vi "Multiply Quaternion by Quaternion.vi"(1 "y":T1, 2 "quaternion":T1) -> (0 "product":T1)   [LabVIEW 2017, in "NI_Kinematics.lvlib"]
doc: "Returns the <B>product</B> of two quaternions or a quaternion and a scalar number. Wire data to the <B>y</B> input to determine the polymorphic instance to use or manually select the instance."
uses:
  <vilib>/robotics/Kinematics/NI_Kinematics.lvlib
  <vilib>/robotics/Kinematics/Quaternion.ctl
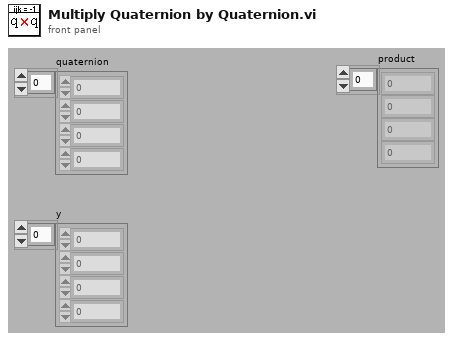
[diagram p1: front panel]
types:
  T1 = typedef "NI_Kinematics.lvlib/Quaternion.ctl" = dbl[]
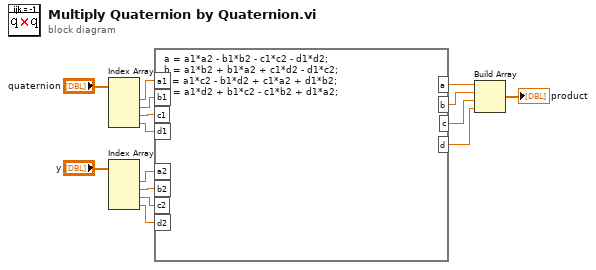
[diagram p0: block diagram]
diagram:
  n1 = Index Array(array="quaternion") -> (element #1=w9:dbl, element #2=w8:dbl, element #3=w7:dbl, element #4=w6:dbl)  [unwired: 4 in]
  n2 = Index Array(array="y") -> (element #1=w4:dbl, element #2=w3:dbl, element #3=w2:dbl, element #4=w1:dbl)  [unwired: 4 in]
  n3 = formula code="a = a1*a2 - b1*b2 - c1*c2 - d1*d2;\nb = a1*b2 + b1*a2 + c1*d2 - d1*c2;\nc = a1*c2 - b1*d2 + c1*a2 + d1*b2;\nd = a1*d2 + b1*c2 - c1*b2 + d1*a2;"("a1"=w9, "b1"=w8, "c1"=w7, "d1"=w6, "a2"=w4, "b2"=w3, "c2"=w2, "d2"=w1) -> ("a"=w14:dbl, "b"=w13:dbl, "c"=w12:dbl, "d"=w11:dbl)
  n4 = Build Array(w14, w13, w12, w11) -> (→"product":dbl[])
